vi "Close.vi"(8 "error in (no error)":errorcluster, 11 "Test Log in":refnum<class "OperationsLog.lvclass">) -> (0 "error out":errorcluster, 3 "Test Log out":refnum<class "OperationsLog.lvclass">)   [LabVIEW 2016, in "OperationsLog.lvclass"]
uses:
  OperationsLog.lvclass
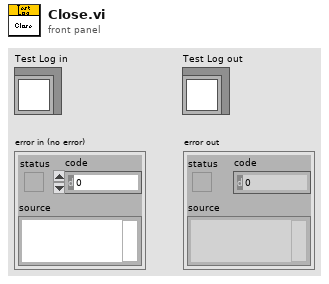
[diagram p1: front panel]
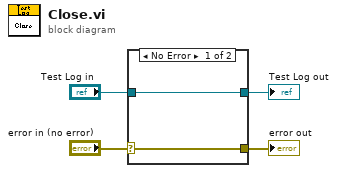
[diagram p0: block diagram]
diagram:
  n1 = case shown="No Error" "error in (no error)" {
    selector: "error in (no error)" -> [w5 w8]
    tunnel: [w5 w8] -> w3
    tunnel: [w6 w7] -> w1
    tunnel: "Test Log in" -> [w6 w7]
    frame No Error {
    }
    frame Error {
    }
  }
  "error out" <- w3
  "Test Log out" <- w1
